vi "Copy Waveform File.vi"(6 "error in":errorcluster, 9 "dst filename":path=path "C:/5-01-003 Active Electrode Min Max/Copy of Waveform 6 10 mA") -> (0 "error out":errorcluster, 4 "new MD5":string)   [LabVIEW 2010]
doc: "This function copies a waveform file. If the target file already exists, it will be deleted."
panel:
  in  "src filename":path=path "C:/5-01-003 Active Electrode Min Max/Waveform 6 10 mA"
  out "old MD5":string
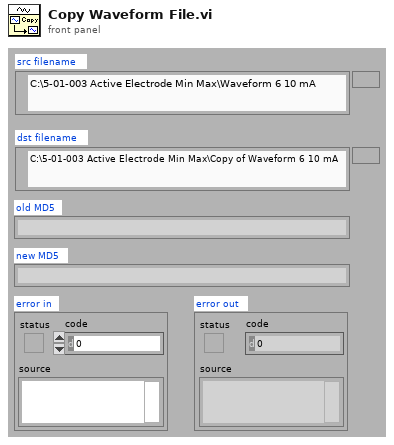
[diagram p1: front panel]
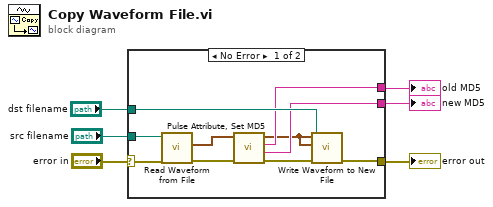
[diagram p0: block diagram]
diagram:
  n1 = case shown="No Error" "error in" {
    selector: "error in" -> [w16 w17]
    tunnel: [w13 w17] -> w5
    tunnel: "src filename" -> [w14 _]
    tunnel: [w9 _] -> w4
    tunnel: [w8 _] -> w2
    tunnel: "dst filename" -> [w10 _]
    frame No Error {
      n2 = call <vilib>:"Read Waveform from File.vi"("error in (no error)"=w16, "file path (dialog if empty)"=w14) -> ("error out"=w12:errorcluster, "first waveform in record"=w11:waveform(dbl))  [unwired: 4 in, 2 out]
      n3 = call "Pulse Attribute, Set MD5.vi"("error in"=w12, "waveform"=w11) -> ("error out"=w15:errorcluster, "New MD5"=w8:string, "Old MD5"=w9:string, "waveform out"=w7:waveform(dbl))  [unwired: 3 in, 1 out]
      n4 = call "Write Waveform to New File.vi"("filepath"=w10, "error in"=w15, "prc waveform"=w7, "raw waveform"=w7) -> ("error out"=w13:errorcluster)  [unwired: 2 in, 3 out]
    }
    frame Error {
    }
  }
  "error out" <- w5
  "new MD5" <- w2
  "old MD5" <- w4
